vi "Write Hardware Handles to Execution Units.vi"(5 "hardware handles":T6, 6 "error in":errorcluster, 9 "RTStateVariables in":T1 {"Inline Execution Units"."Outgoing Data References"."Data Reference" format="%.0x"; "Inline Execution Units"."Incoming Data References" format="%.0x"}) -> (0 "error out":errorcluster, 3 "RTStateVariables out":T1 {"Inline Execution Units"."Outgoing Data References"."Data Reference" format="%.0x"; "Inline Execution Units"."Incoming Data References" format="%.0x"})   [LabVIEW 2020, in "Ballard ARINC 429 Engine.lvlib" / "Custom Device.lvlib"]
uses:
  Custom Device.lvlib
  Hardware Handles.ctl
  RTStateVariables.ctl
  <vilib>/NI/NIVS Inline Async API/_VS Inline Async API/VS Inline Async API/VS Inline Async API.lvclass
  Inline Execution Unit Runtime Information.ctl
  <vilib>/NI VeriStand/Custom Device API/Data Reference.ctl
  <vilib>/NI VeriStand/Custom Device API/Block Data Reference.ctl
  Asynchronous Execution Unit Runtime Information.ctl
  Implementation/Ballard ARINC-429 Execution Unit/Ballard ARINC-429 Execution Unit.lvclass
  C:/Git/niveristand-ballard-arinc429-custom-device/Source/Custom Device Support/Engine/Interfaces/Execution Unit/Execution Unit.lvclass
  Implementation/Ballard ARINC-429 Execution Unit/Ballard ARINC-429 Execution Unit.lvclass/Ballard ARINC-429 Execution Unit.ctl
  Interfaces/Execution Unit/Execution Unit.lvclass
  <vilib>/NI VeriStand/Custom Device API/Custom Device API.lvlib
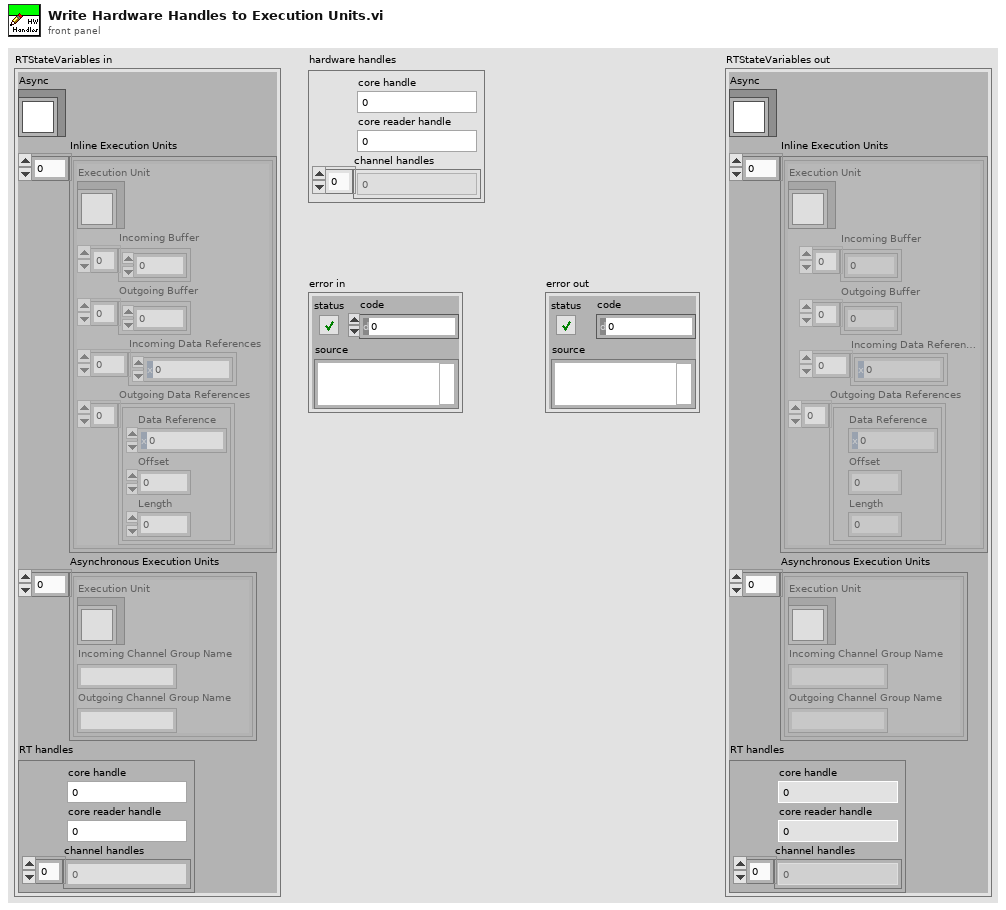
[diagram p1: front panel]
types:
  T1 = typedef "Ballard ARINC 429 Engine.lvlib/Custom Device.lvlib/RTStateVariables.ctl" = cluster{"Async":refnum<class "VS Inline Async API.lvclass">, "Inline Execution Units":T2[], "Asynchronous Execution Units":T5[], "RT handles":T6}
  T2 = typedef "Ballard ARINC 429 Engine.lvlib/Custom Device.lvlib/Inline Execution Unit Runtime Information.ctl" = cluster{"Execution Unit":refnum<class "Execution Unit.lvclass">, "Incoming Buffer":dbl[], "Outgoing Buffer":dbl[], "Incoming Data References":T3[], "Outgoing Data References":T4[]}
  T3 = typedef "Custom Device API.lvlib/Data Reference.ctl" = i32
  T4 = typedef "Custom Device API.lvlib/Block Data Reference.ctl" = cluster{"Data Reference":T3, "Offset":u64, "Length":u64}
  T5 = typedef "Ballard ARINC 429 Engine.lvlib/Custom Device.lvlib/Asynchronous Execution Unit Runtime Information.ctl" = cluster{"Execution Unit":refnum<class "Execution Unit.lvclass">, "Incoming Channel Group Name":string, "Outgoing Channel Group Name":string}
  T6 = typedef "Ballard ARINC 429 Engine.lvlib/Custom Device.lvlib/Hardware Handles.ctl" = cluster{"core handle":u64, "core reader handle":u64, "channel handles":u64[]}
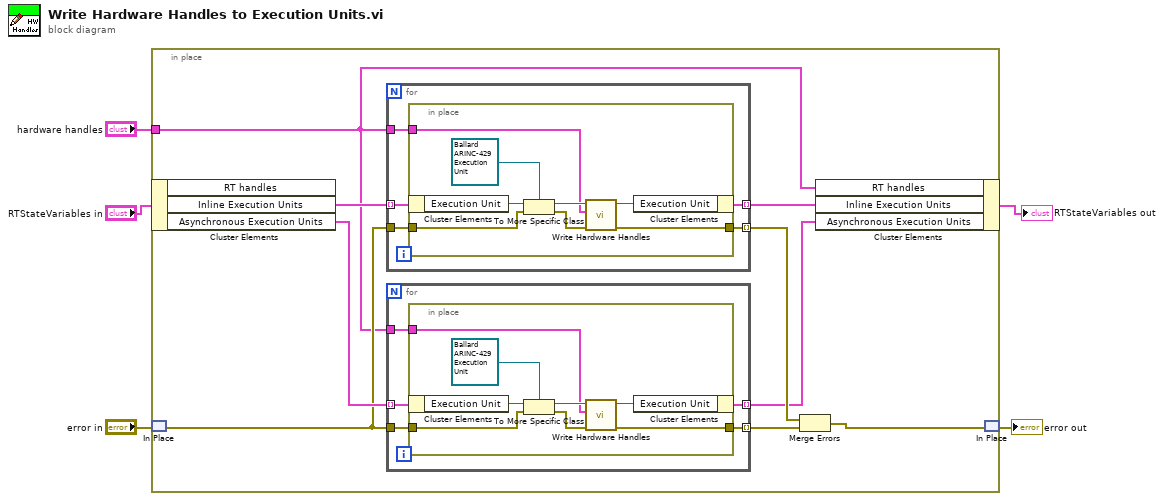
[diagram p0: block diagram]
diagram:
  n1 = in-place {
    in-place-border: "hardware handles" -> [w6]
    n2 = in-place-cluster #1("RTStateVariables in") -> ("Inline Execution Units"=w12:T2[], "Asynchronous Execution Units"=w11:T5[])  [unwired: 1 out]
    n3 = in-place-match #2("error in") -> (w8:errorcluster)
    n4 = for {
      tunnel: w12 -> [w31] mode=indexing
      tunnel: w6 -> [w32]
      tunnel: [w30] -> w10 mode=indexing
      tunnel: [w29] -> w14 mode=indexing
      tunnel: w8 -> [w28]
      n5 = in-place {
        in-place-border: w32 -> [w37]
        in-place-border: [w34] -> w29
        in-place-border: w28 -> [w33]
        n6 = in-place-cluster #3(w31) -> ("Execution Unit"=w36:refnum<class "Execution Unit.lvclass">)
        n7 = To More Specific Class(target class=refnum<class "Ballard ARINC-429 Execution Unit.lvclass"> refnum ("Ballard ARINC-429 Execution Unit in"), reference=w36, error in=w33) -> (specific class reference=w39:refnum<class "Ballard ARINC-429 Execution Unit.lvclass">, error out=w38:errorcluster)
        n8 = call "Write Hardware Handles.vi"("error in"=w38, "hardware handles"=w37, "Ballard ARINC-429 Execution Unit in"=w39) -> ("error out"=w34:errorcluster, "Ballard ARINC-429 Execution Unit out"=w35:refnum<class "Ballard ARINC-429 Execution Unit.lvclass">)  [unwired: 7 in]
        n9 = in-place-cluster #3("Execution Unit"=w35) -> (w30:T2)
      }
    }
    n10 = for {
      tunnel: w11 -> [w18] mode=indexing
      tunnel: w6 -> [w19]
      tunnel: [w17] -> w9 mode=indexing
      tunnel: [w16] -> w13 mode=indexing
      tunnel: w8 -> [w15]
      n11 = in-place {
        in-place-border: w19 -> [w24]
        in-place-border: [w21] -> w16
        in-place-border: w15 -> [w20]
        n12 = in-place-cluster #4(w18) -> ("Execution Unit"=w23:refnum<class "Execution Unit.lvclass">)
        n13 = To More Specific Class(target class=refnum<class "Ballard ARINC-429 Execution Unit.lvclass"> refnum ("Ballard ARINC-429 Execution Unit in"), reference=w23, error in=w20) -> (specific class reference=w26:refnum<class "Ballard ARINC-429 Execution Unit.lvclass">, error out=w25:errorcluster)
        n14 = call "Write Hardware Handles.vi"("error in"=w25, "hardware handles"=w24, "Ballard ARINC-429 Execution Unit in"=w26) -> ("error out"=w21:errorcluster, "Ballard ARINC-429 Execution Unit out"=w22:refnum<class "Ballard ARINC-429 Execution Unit.lvclass">)  [unwired: 7 in]
        n15 = in-place-cluster #4("Execution Unit"=w22) -> (w17:T5)
      }
    }
    n16 = Merge Errors(w14, w13) -> (w7:errorcluster)
    n17 = in-place-cluster #1("RT handles"=w6, "Inline Execution Units"=w10, "Asynchronous Execution Units"=w9) -> (→"RTStateVariables out":T1)
    n18 = in-place-match #2(w7) -> (→"error out":errorcluster)
  }
